vi "Minimal X410 (FPGA).vi"() -> ()   [LabVIEW 2023]
uses:
  <vilib>/Platform/TimedLoop/XDataNode/XDataNode.xnode
  <vilib>/Platform/TimedLoop/XDataNode/nitl_modes.ctl
  <vilib>/Platform/TimedLoop/XDataNode/XDNodeRunTimeDep.lvlib
  <vilib>/Platform/TimedLoop/XDataNode/wakeup.ctl
  <vilib>/Platform/TimedLoop/XDataNode/timing_clust.ctl
  <vilib>/eio/EIONode/EIONode.xnode
  <vilib>/rvi/eio/common/nirviEmuTemplateMethod_errors.vi
  <instrlib>/_niInstr/DSP/v1/Shared/Public/IQ Data.ctl
  <instrlib>/_niInstr/DSP/v1/FPGA/Public/Sub VIs/Data Conversion/I16 to IQ - 1 spc - S18.1.vi
  <instrlib>/niUSRP/Reference FPGA/Tx Core/niUSRP Tx Core v1 FPGA.lvclass
  <vilib>/rvi/DataTransferAndStorage/Container/XNode/niFpgaContainer.xnode
  <vilib>/rvi/FIFO/Fifo_Resource/niFpgaFifoEmulationRefIn.vi
panel:
  out "scratch reg value":u32
  in  "update scratch reg":bool
  in  "scratch reg new value":u32
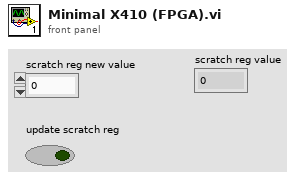
[diagram p1: front panel]
types:
  T1 = typedef "XDNodeRunTimeDep.lvlib/timing_clust.ctl" = cluster{"Expected End [f-1]":u64, "Actual End [f-1]":u64, "Finished Late? [f-1]":bool, "Expected End [i-1]":u64, "Actual End [i-1]":u64, "Finished Late? [i-1]":bool, "Expected Start [i]":u64, "Actual Start [i]":u64, "Expected Start [f]":u64, "Actual Start [f]":u64, "Source Name":string, "Structure Name":string, "Period":i64, "Deadline":i64, "Offset":i64, "Start":i64, "Priority":i32, "Timeout":i32, "Mode":T2, "Wakeup Reason":T3, "Error":errorcluster, "Source Type":string, "Secondary Source Type":string, "Global End Time":u64, "Global Start Time":u64, "Frame Duration":u64, "Iteration Duration":u64, "Assigned CPU":i32, "I/O Scan Engine Mode":u32}
  T2 = typedef "XDNodeRunTimeDep.lvlib/nitl_modes.ctl" = enum32{"No Change", "Process missed periods, maintain original phase", "Discard missed periods, maintain original phase", "Process missed periods, ignore original phase", "Discard missed periods, ignore original phase"}
  T3 = typedef "XDNodeRunTimeDep.lvlib/wakeup.ctl" = enum32{"Normal", "Aborted", "Asynchronous wakeup", "Timing source error", "Timed loop error", "Timeout"}
  T4 = typedef "niInstr DSP v1 Shared.lvlib/IQ Data.ctl" = cluster{"I":fxp<+/-,18,1>, "Q":fxp<+/-,18,1>, "overflow":bool}
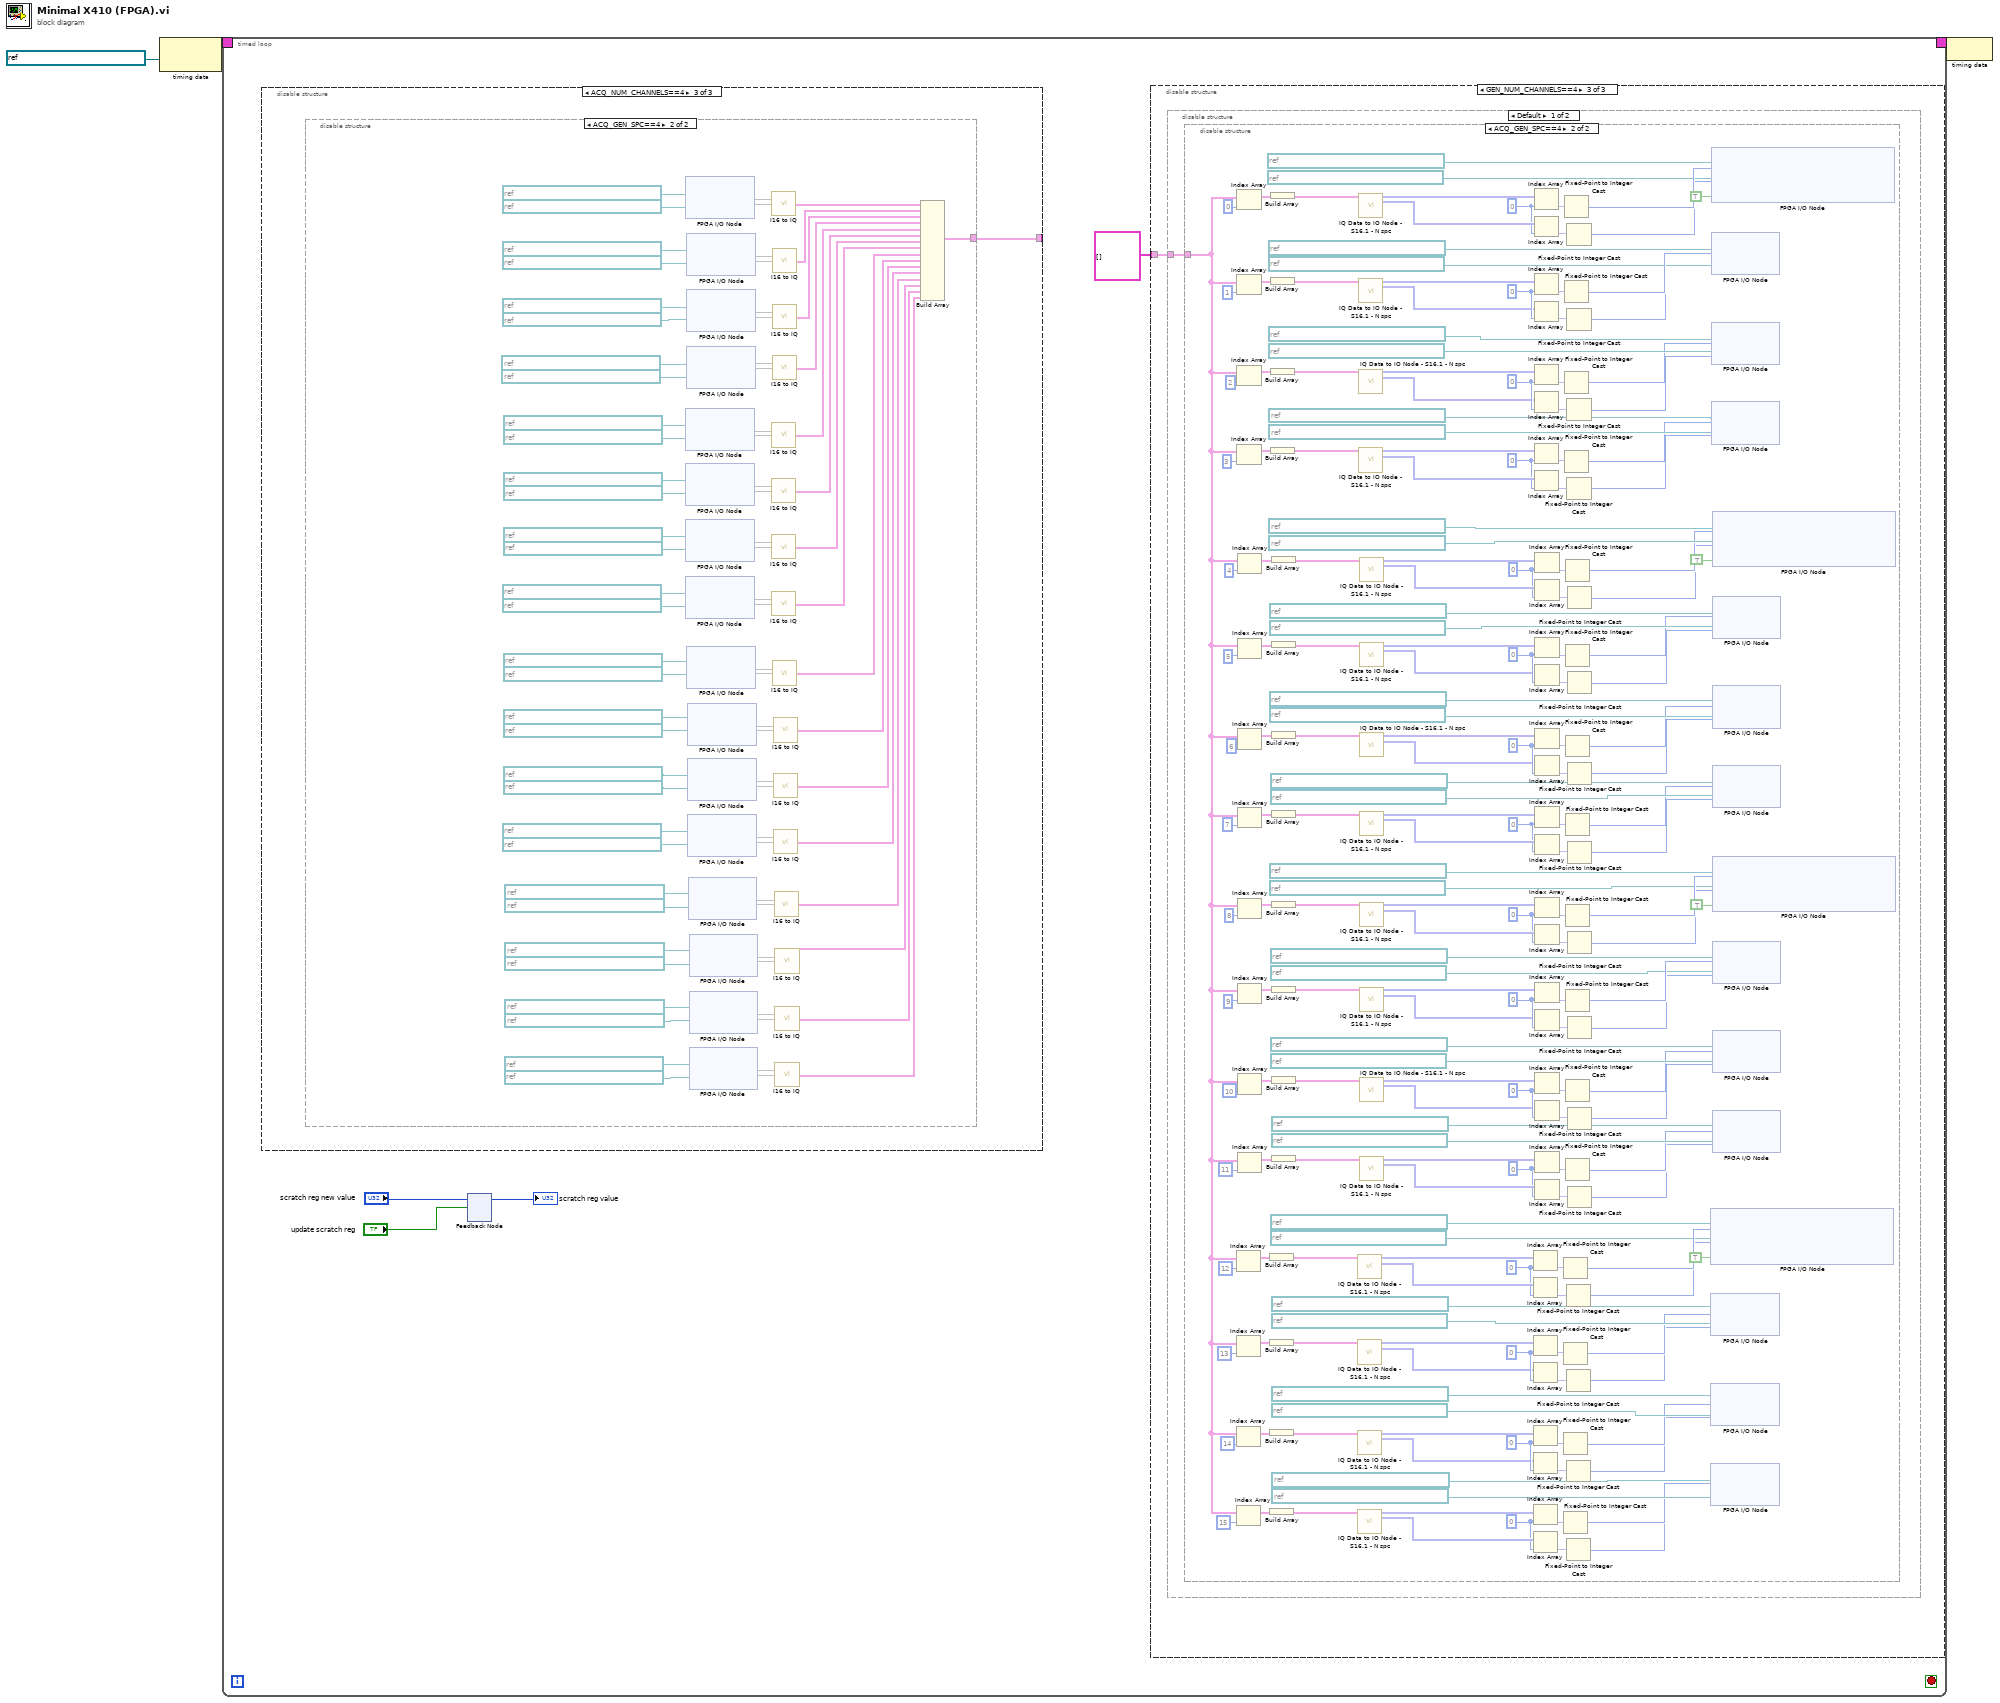
[diagram p0: block diagram]
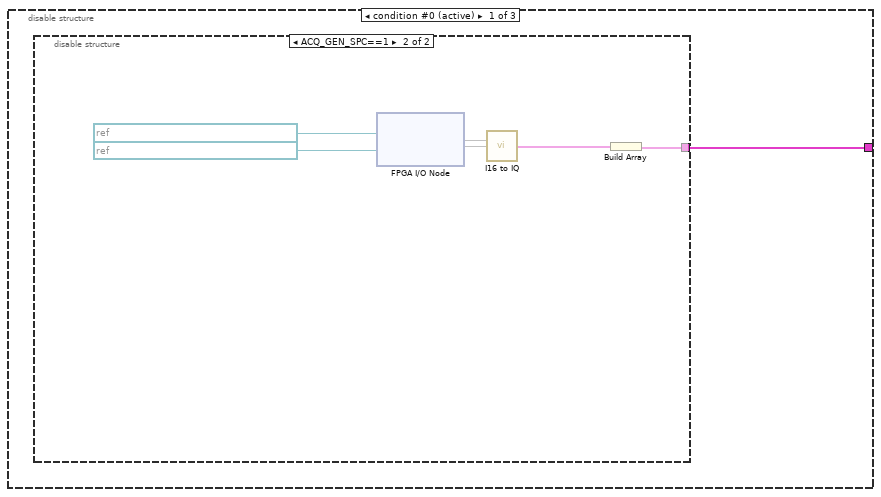
[diagram p2: hidden frame]
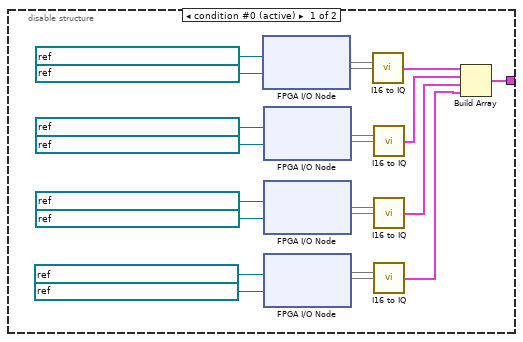
[diagram p3: hidden frame]
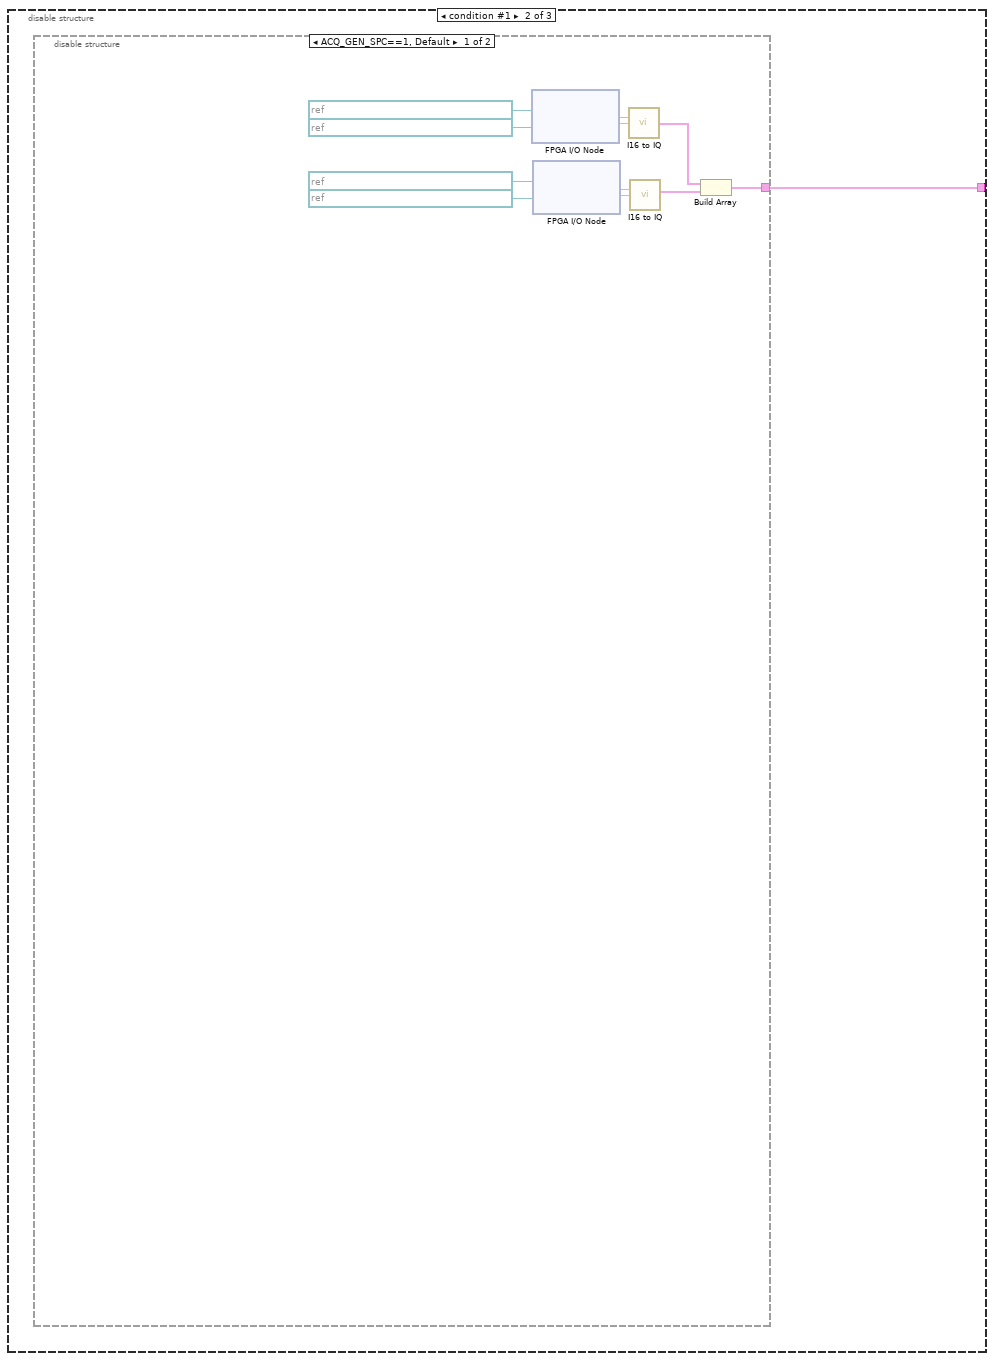
[diagram p4: hidden frame]
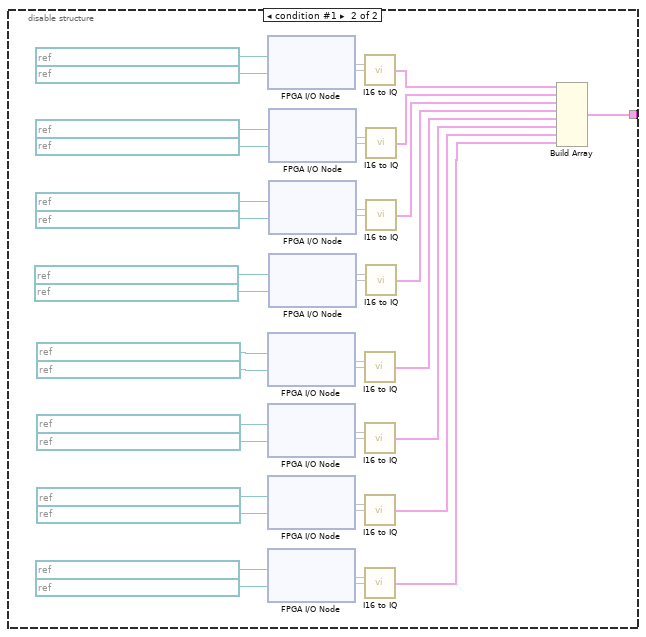
[diagram p5: hidden frame]
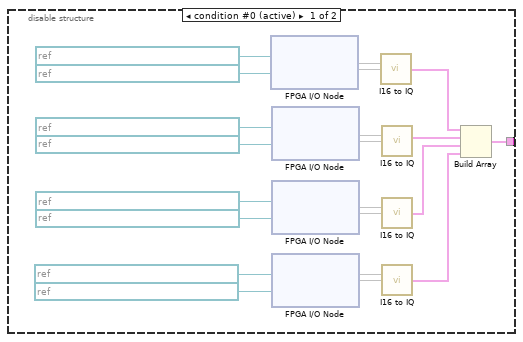
[diagram p6: hidden frame]
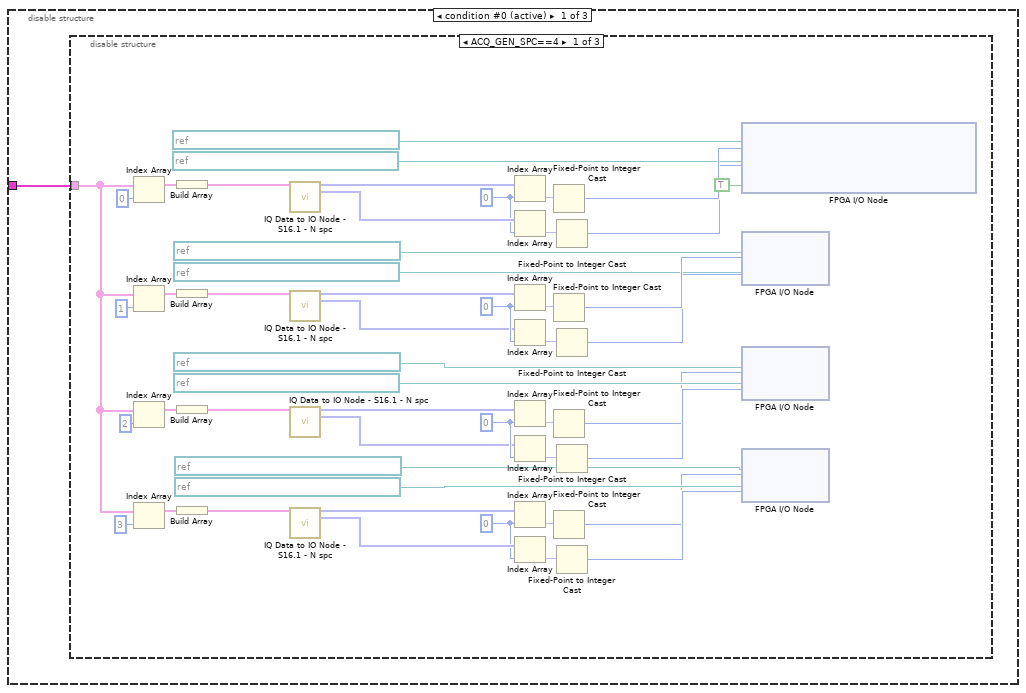
[diagram p7: hidden frame]
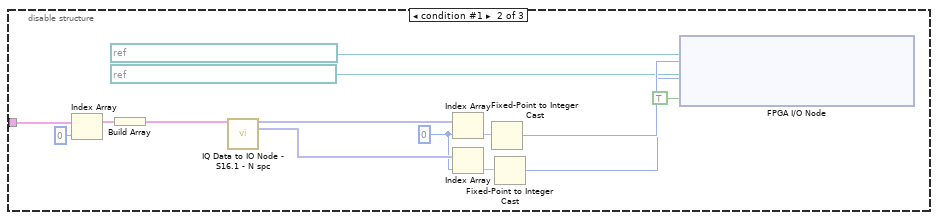
[diagram p8: hidden frame]
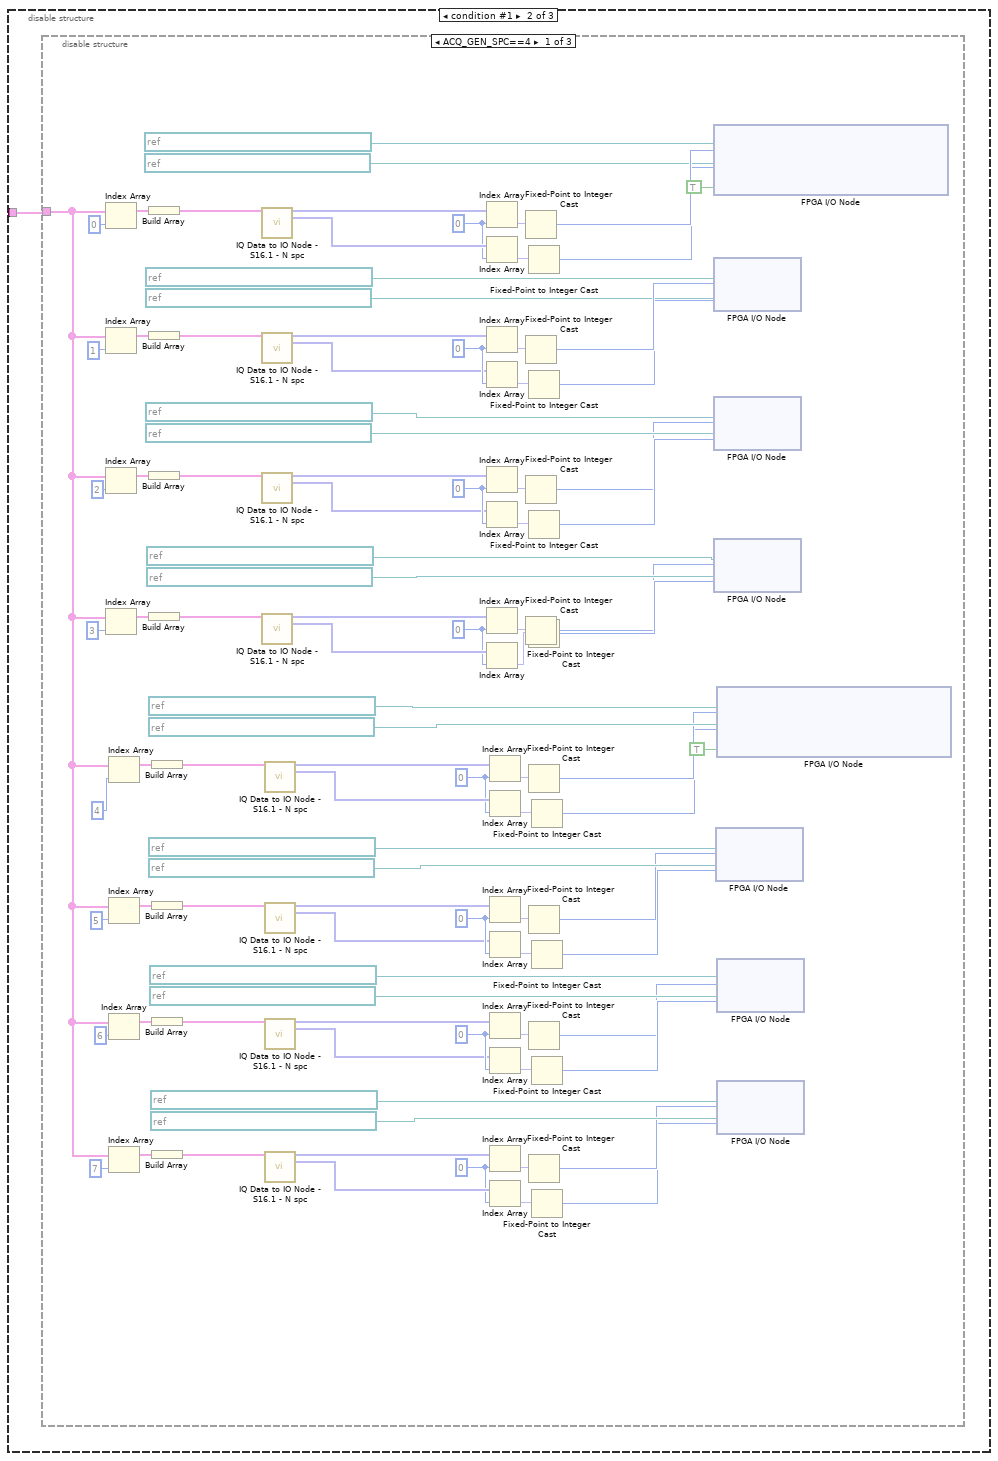
[diagram p10: hidden frame]
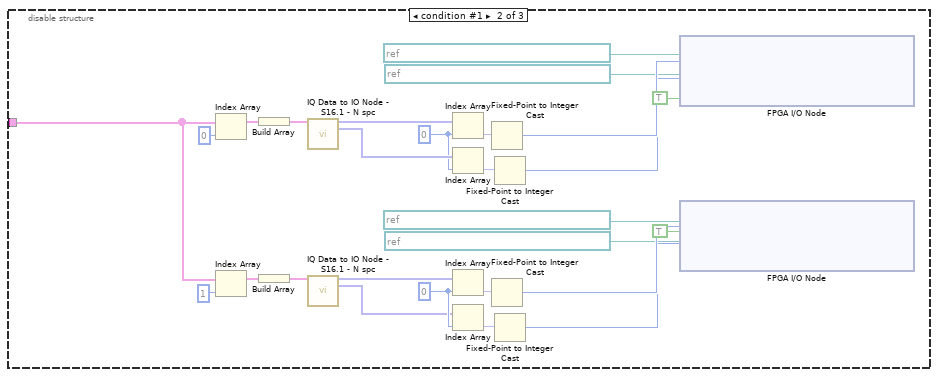
[diagram p11: hidden frame]
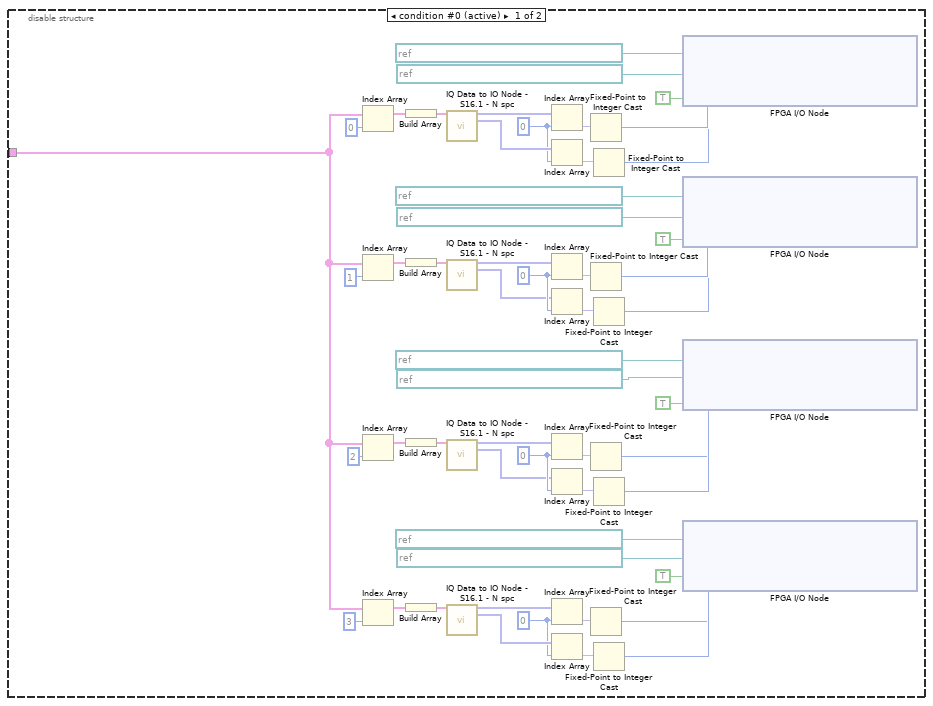
[diagram p13: hidden frame]
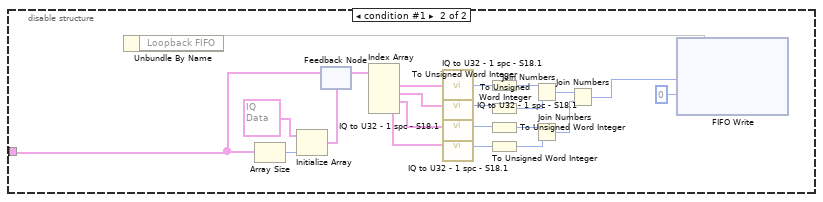
[diagram p14: hidden frame]
diagram:
  n1 = node-c288(refnum<k21> "Daughterboard 0\\Data Clock" ("Source Name")) -> (w3:T1)
  n2 = timed-loop {
    timing: w3 -> [_]
    timing-out: [_] -> w2
    stop <- _ stop-if-true
    n3 = disable-structure shown="ACQ_NUM_CHANNELS==4" {
      disable-tunnel: [w8 w36 w89] -> _
      frame condition #0 (active) {
        n4 = disable-structure shown="ACQ_GEN_SPC==1" {
          disable-tunnel: [w9 w35] -> w8
          frame condition #0 (active) {
            n5 = xnode "FPGA I/O Node"("FPGA I/O In"=refnum<k21> "Daughterboard 0\\RF 0\\Rx\\I0", "FPGA I/O In"=refnum<k21> "Daughterboard 0\\RF 0\\Rx\\Q0") -> ("I/O Item"=w29, "I/O Item"=w28)  [unwired: 2 out]
            n6 = xnode "FPGA I/O Node"("FPGA I/O In"=refnum<k21> "Daughterboard 0\\RF 0\\Rx\\I1", "FPGA I/O In"=refnum<k21> "Daughterboard 0\\RF 0\\Rx\\Q1") -> ("I/O Item"=w27, "I/O Item"=w26)  [unwired: 2 out]
            n7 = xnode "FPGA I/O Node"("FPGA I/O In"=refnum<k21> "Daughterboard 0\\RF 0\\Rx\\I2", "FPGA I/O In"=refnum<k21> "Daughterboard 0\\RF 0\\Rx\\Q2") -> ("I/O Item"=w25, "I/O Item"=w24)  [unwired: 2 out]
            n8 = xnode "FPGA I/O Node"("FPGA I/O In"=refnum<k21> "Daughterboard 0\\RF 0\\Rx\\I3", "FPGA I/O In"=refnum<k21> "Daughterboard 0\\RF 0\\Rx\\Q3") -> ("I/O Item"=w23, "I/O Item"=w22)  [unwired: 2 out]
            n9 = call-poly <instrlib>:"I16 to IQ.vi"("I"=w29, "Q"=w28) -> ("IQ"=w13:T4)  [unwired: 13 in]
            n10 = call-poly <instrlib>:"I16 to IQ.vi"("I"=w27, "Q"=w26) -> ("IQ"=w12:T4)  [unwired: 13 in]
            n11 = call-poly <instrlib>:"I16 to IQ.vi"("I"=w25, "Q"=w24) -> ("IQ"=w11:T4)  [unwired: 13 in]
            n12 = call-poly <instrlib>:"I16 to IQ.vi"("I"=w23, "Q"=w22) -> ("IQ"=w10:T4)  [unwired: 13 in]
            n13 = Build Array(w13, w12, w11, w10) -> (w9:T4[])
          }
          frame condition #1 {
            n14 = xnode "FPGA I/O Node"("FPGA I/O In"=refnum<k21> "Daughterboard 0\\RF 0\\Rx\\I", "FPGA I/O In"=refnum<k21> "Daughterboard 0\\RF 0\\Rx\\Q") -> ("I/O Item"=w34, "I/O Item"=w33)  [unwired: 2 out]
            n15 = call-poly <instrlib>:"I16 to IQ.vi"("I"=w34, "Q"=w33) -> ("IQ"=w30:T4)  [unwired: 13 in]
            n16 = Build Array(w30) -> (w35:T4[])
          }
        }
      }
      frame condition #1 {
        n17 = disable-structure shown="ACQ_GEN_SPC==1, Default" {
          disable-tunnel: [w37 w88] -> w36
          frame condition #0 (active) {
            n18 = xnode "FPGA I/O Node"("FPGA I/O In"=refnum<k21> "Daughterboard 0\\RF 0\\Rx\\I", "FPGA I/O In"=refnum<k21> "Daughterboard 0\\RF 0\\Rx\\Q") -> ("I/O Item"=w47, "I/O Item"=w46)  [unwired: 2 out]
            n19 = xnode "FPGA I/O Node"("FPGA I/O In"=refnum<k21> "Daughterboard 0\\RF 1\\Rx\\I", "FPGA I/O In"=refnum<k21> "Daughterboard 0\\RF 1\\Rx\\Q") -> ("I/O Item"=w45, "I/O Item"=w44)  [unwired: 2 out]
            n20 = call-poly <instrlib>:"I16 to IQ.vi"("I"=w47, "Q"=w46) -> ("IQ"=w39:T4)  [unwired: 13 in]
            n21 = call-poly <instrlib>:"I16 to IQ.vi"("I"=w45, "Q"=w44) -> ("IQ"=w38:T4)  [unwired: 13 in]
            n22 = Build Array(w39, w38) -> (w37:T4[])
          }
          frame condition #1 {
            n23 = xnode "FPGA I/O Node"("FPGA I/O In"=refnum<k21> "Daughterboard 0\\RF 0\\Rx\\I0", "FPGA I/O In"=refnum<k21> "Daughterboard 0\\RF 0\\Rx\\Q0") -> ("I/O Item"=w87, "I/O Item"=w86)  [unwired: 2 out]
            n24 = xnode "FPGA I/O Node"("FPGA I/O In"=refnum<k21> "Daughterboard 0\\RF 1\\Rx\\I0", "FPGA I/O In"=refnum<k21> "Daughterboard 0\\RF 1\\Rx\\Q0") -> ("I/O Item"=w78, "I/O Item"=w77)  [unwired: 2 out]
            n25 = xnode "FPGA I/O Node"("FPGA I/O In"=refnum<k21> "Daughterboard 0\\RF 1\\Rx\\I1", "FPGA I/O In"=refnum<k21> "Daughterboard 0\\RF 1\\Rx\\Q1") -> ("I/O Item"=w75, "I/O Item"=w74)  [unwired: 2 out]
            n26 = xnode "FPGA I/O Node"("FPGA I/O In"=refnum<k21> "Daughterboard 0\\RF 0\\Rx\\I2", "FPGA I/O In"=refnum<k21> "Daughterboard 0\\RF 1\\Rx\\Q2") -> ("I/O Item"=w73, "I/O Item"=w72)  [unwired: 2 out]
            n27 = xnode "FPGA I/O Node"("FPGA I/O In"=refnum<k21> "Daughterboard 0\\RF 1\\Rx\\I3", "FPGA I/O In"=refnum<k21> "Daughterboard 0\\RF 1\\Rx\\Q3") -> ("I/O Item"=w71, "I/O Item"=w70)  [unwired: 2 out]
            n28 = xnode "FPGA I/O Node"("FPGA I/O In"=refnum<k21> "Daughterboard 0\\RF 0\\Rx\\I1", "FPGA I/O In"=refnum<k21> "Daughterboard 0\\RF 0\\Rx\\Q1") -> ("I/O Item"=w84, "I/O Item"=w83)  [unwired: 2 out]
            n29 = xnode "FPGA I/O Node"("FPGA I/O In"=refnum<k21> "Daughterboard 0\\RF 0\\Rx\\I2", "FPGA I/O In"=refnum<k21> "Daughterboard 0\\RF 0\\Rx\\Q2") -> ("I/O Item"=w82, "I/O Item"=w81)  [unwired: 2 out]
            n30 = xnode "FPGA I/O Node"("FPGA I/O In"=refnum<k21> "Daughterboard 0\\RF 0\\Rx\\I3", "FPGA I/O In"=refnum<k21> "Daughterboard 0\\RF 0\\Rx\\Q3") -> ("I/O Item"=w80, "I/O Item"=w79)  [unwired: 2 out]
            n31 = call-poly <instrlib>:"I16 to IQ.vi"("I"=w87, "Q"=w86) -> ("IQ"=w85:T4)  [unwired: 13 in]
            n32 = call-poly <instrlib>:"I16 to IQ.vi"("I"=w78, "Q"=w77) -> ("IQ"=w76:T4)  [unwired: 13 in]
            n33 = call-poly <instrlib>:"I16 to IQ.vi"("I"=w75, "Q"=w74) -> ("IQ"=w66:T4)  [unwired: 13 in]
            n34 = call-poly <instrlib>:"I16 to IQ.vi"("I"=w73, "Q"=w72) -> ("IQ"=w65:T4)  [unwired: 13 in]
            n35 = call-poly <instrlib>:"I16 to IQ.vi"("I"=w71, "Q"=w70) -> ("IQ"=w64:T4)  [unwired: 13 in]
            n36 = call-poly <instrlib>:"I16 to IQ.vi"("I"=w84, "Q"=w83) -> ("IQ"=w69:T4)  [unwired: 13 in]
            n37 = call-poly <instrlib>:"I16 to IQ.vi"("I"=w82, "Q"=w81) -> ("IQ"=w68:T4)  [unwired: 13 in]
            n38 = call-poly <instrlib>:"I16 to IQ.vi"("I"=w80, "Q"=w79) -> ("IQ"=w67:T4)  [unwired: 13 in]
            n39 = Build Array(w85, w69, w68, w67, w76, w66, w65, w64) -> (w88:T4[])
          }
        }
      }
      frame condition #2 {
        n40 = disable-structure shown="ACQ_GEN_SPC==4" {
          disable-tunnel: [w90 w191] -> w89
          frame condition #0 (active) {
            n41 = xnode "FPGA I/O Node"("FPGA I/O In"=refnum<k21> "Daughterboard 0\\RF 0\\Rx\\I", "FPGA I/O In"=refnum<k21> "Daughterboard 0\\RF 0\\Rx\\Q") -> ("I/O Item"=w110, "I/O Item"=w109)  [unwired: 2 out]
            n42 = xnode "FPGA I/O Node"("FPGA I/O In"=refnum<k21> "Daughterboard 0\\RF 1\\Rx\\I", "FPGA I/O In"=refnum<k21> "Daughterboard 0\\RF 1\\Rx\\Q") -> ("I/O Item"=w108, "I/O Item"=w107)  [unwired: 2 out]
            n43 = xnode "FPGA I/O Node"("FPGA I/O In"=refnum<k21> "Daughterboard 1\\RF 0\\Rx\\I", "FPGA I/O In"=refnum<k21> "Daughterboard 1\\RF 0\\Rx\\Q") -> ("I/O Item"=w106, "I/O Item"=w105)  [unwired: 2 out]
            n44 = xnode "FPGA I/O Node"("FPGA I/O In"=refnum<k21> "Daughterboard 1\\RF 1\\Rx\\I", "FPGA I/O In"=refnum<k21> "Daughterboard 1\\RF 1\\Rx\\Q") -> ("I/O Item"=w104, "I/O Item"=w103)  [unwired: 2 out]
            n45 = call-poly <instrlib>:"I16 to IQ.vi"("I"=w110, "Q"=w109) -> ("IQ"=w94:T4)  [unwired: 13 in]
            n46 = call-poly <instrlib>:"I16 to IQ.vi"("I"=w108, "Q"=w107) -> ("IQ"=w93:T4)  [unwired: 13 in]
            n47 = call-poly <instrlib>:"I16 to IQ.vi"("I"=w106, "Q"=w105) -> ("IQ"=w92:T4)  [unwired: 13 in]
            n48 = call-poly <instrlib>:"I16 to IQ.vi"("I"=w104, "Q"=w103) -> ("IQ"=w91:T4)  [unwired: 13 in]
            n49 = Build Array(w94, w93, w92, w91) -> (w90:T4[])
          }
          frame condition #1 {
            n50 = xnode "FPGA I/O Node"("FPGA I/O In"=refnum<k21> "Daughterboard 0\\RF 0\\Rx\\I0", "FPGA I/O In"=refnum<k21> "Daughterboard 0\\RF 0\\Rx\\Q0") -> ("I/O Item"=w190, "I/O Item"=w189)  [unwired: 2 out]
            n51 = xnode "FPGA I/O Node"("FPGA I/O In"=refnum<k21> "Daughterboard 0\\RF 1\\Rx\\I0", "FPGA I/O In"=refnum<k21> "Daughterboard 0\\RF 1\\Rx\\Q0") -> ("I/O Item"=w181, "I/O Item"=w180)  [unwired: 2 out]
            n52 = xnode "FPGA I/O Node"("FPGA I/O In"=refnum<k21> "Daughterboard 0\\RF 1\\Rx\\I1", "FPGA I/O In"=refnum<k21> "Daughterboard 0\\RF 1\\Rx\\Q1") -> ("I/O Item"=w178, "I/O Item"=w177)  [unwired: 2 out]
            n53 = xnode "FPGA I/O Node"("FPGA I/O In"=refnum<k21> "Daughterboard 0\\RF 1\\Rx\\I2", "FPGA I/O In"=refnum<k21> "Daughterboard 0\\RF 1\\Rx\\Q2") -> ("I/O Item"=w176, "I/O Item"=w175)  [unwired: 2 out]
            n54 = xnode "FPGA I/O Node"("FPGA I/O In"=refnum<k21> "Daughterboard 0\\RF 1\\Rx\\I3", "FPGA I/O In"=refnum<k21> "Daughterboard 0\\RF 1\\Rx\\Q3") -> ("I/O Item"=w174, "I/O Item"=w173)  [unwired: 2 out]
            n55 = xnode "FPGA I/O Node"("FPGA I/O In"=refnum<k21> "Daughterboard 0\\RF 0\\Rx\\I1", "FPGA I/O In"=refnum<k21> "Daughterboard 0\\RF 0\\Rx\\Q1") -> ("I/O Item"=w187, "I/O Item"=w186)  [unwired: 2 out]
            n56 = xnode "FPGA I/O Node"("FPGA I/O In"=refnum<k21> "Daughterboard 0\\RF 0\\Rx\\I2", "FPGA I/O In"=refnum<k21> "Daughterboard 0\\RF 0\\Rx\\Q2") -> ("I/O Item"=w185, "I/O Item"=w184)  [unwired: 2 out]
            n57 = xnode "FPGA I/O Node"("FPGA I/O In"=refnum<k21> "Daughterboard 0\\RF 0\\Rx\\I3", "FPGA I/O In"=refnum<k21> "Daughterboard 0\\RF 0\\Rx\\Q3") -> ("I/O Item"=w183, "I/O Item"=w182)  [unwired: 2 out]
            n58 = xnode "FPGA I/O Node"("FPGA I/O In"=refnum<k21> "Daughterboard 1\\RF 0\\Rx\\I0", "FPGA I/O In"=refnum<k21> "Daughterboard 1\\RF 0\\Rx\\Q0") -> ("I/O Item"=w172, "I/O Item"=w171)  [unwired: 2 out]
            n59 = xnode "FPGA I/O Node"("FPGA I/O In"=refnum<k21> "Daughterboard 1\\RF 0\\Rx\\I1", "FPGA I/O In"=refnum<k21> "Daughterboard 1\\RF 0\\Rx\\Q1") -> ("I/O Item"=w170, "I/O Item"=w169)  [unwired: 2 out]
            n60 = xnode "FPGA I/O Node"("FPGA I/O In"=refnum<k21> "Daughterboard 1\\RF 0\\Rx\\I2", "FPGA I/O In"=refnum<k21> "Daughterboard 1\\RF 0\\Rx\\Q2") -> ("I/O Item"=w168, "I/O Item"=w167)  [unwired: 2 out]
            n61 = xnode "FPGA I/O Node"("FPGA I/O In"=refnum<k21> "Daughterboard 1\\RF 0\\Rx\\I3", "FPGA I/O In"=refnum<k21> "Daughterboard 1\\RF 0\\Rx\\Q3") -> ("I/O Item"=w166, "I/O Item"=w165)  [unwired: 2 out]
            n62 = xnode "FPGA I/O Node"("FPGA I/O In"=refnum<k21> "Daughterboard 1\\RF 1\\Rx\\I0", "FPGA I/O In"=refnum<k21> "Daughterboard 1\\RF 1\\Rx\\Q0") -> ("I/O Item"=w164, "I/O Item"=w163)  [unwired: 2 out]
            n63 = xnode "FPGA I/O Node"("FPGA I/O In"=refnum<k21> "Daughterboard 1\\RF 1\\Rx\\I1", "FPGA I/O In"=refnum<k21> "Daughterboard 1\\RF 1\\Rx\\Q1") -> ("I/O Item"=w162, "I/O Item"=w161)  [unwired: 2 out]
            n64 = xnode "FPGA I/O Node"("FPGA I/O In"=refnum<k21> "Daughterboard 1\\RF 1\\Rx\\I2", "FPGA I/O In"=refnum<k21> "Daughterboard 1\\RF 1\\Rx\\Q2") -> ("I/O Item"=w160, "I/O Item"=w159)  [unwired: 2 out]
            n65 = xnode "FPGA I/O Node"("FPGA I/O In"=refnum<k21> "Daughterboard 1\\RF 1\\Rx\\I3", "FPGA I/O In"=refnum<k21> "Daughterboard 1\\RF 1\\Rx\\Q3") -> ("I/O Item"=w158, "I/O Item"=w140)  [unwired: 2 out]
            n66 = call-poly <instrlib>:"I16 to IQ.vi"("I"=w190, "Q"=w189) -> ("IQ"=w188:T4)  [unwired: 13 in]
            n67 = call-poly <instrlib>:"I16 to IQ.vi"("I"=w181, "Q"=w180) -> ("IQ"=w179:T4)  [unwired: 13 in]
            n68 = call-poly <instrlib>:"I16 to IQ.vi"("I"=w178, "Q"=w177) -> ("IQ"=w153:T4)  [unwired: 13 in]
            n69 = call-poly <instrlib>:"I16 to IQ.vi"("I"=w176, "Q"=w175) -> ("IQ"=w152:T4)  [unwired: 13 in]
            n70 = call-poly <instrlib>:"I16 to IQ.vi"("I"=w174, "Q"=w173) -> ("IQ"=w151:T4)  [unwired: 13 in]
            n71 = call-poly <instrlib>:"I16 to IQ.vi"("I"=w187, "Q"=w186) -> ("IQ"=w156:T4)  [unwired: 13 in]
            n72 = call-poly <instrlib>:"I16 to IQ.vi"("I"=w185, "Q"=w184) -> ("IQ"=w155:T4)  [unwired: 13 in]
            n73 = call-poly <instrlib>:"I16 to IQ.vi"("I"=w183, "Q"=w182) -> ("IQ"=w154:T4)  [unwired: 13 in]
            n74 = call-poly <instrlib>:"I16 to IQ.vi"("I"=w172, "Q"=w171) -> ("IQ"=w157:T4)  [unwired: 13 in]
            n75 = call-poly <instrlib>:"I16 to IQ.vi"("I"=w170, "Q"=w169) -> ("IQ"=w150:T4)  [unwired: 13 in]
            n76 = call-poly <instrlib>:"I16 to IQ.vi"("I"=w168, "Q"=w167) -> ("IQ"=w149:T4)  [unwired: 13 in]
            n77 = call-poly <instrlib>:"I16 to IQ.vi"("I"=w166, "Q"=w165) -> ("IQ"=w148:T4)  [unwired: 13 in]
            n78 = call-poly <instrlib>:"I16 to IQ.vi"("I"=w164, "Q"=w163) -> ("IQ"=w147:T4)  [unwired: 13 in]
            n79 = call-poly <instrlib>:"I16 to IQ.vi"("I"=w162, "Q"=w161) -> ("IQ"=w146:T4)  [unwired: 13 in]
            n80 = call-poly <instrlib>:"I16 to IQ.vi"("I"=w160, "Q"=w159) -> ("IQ"=w145:T4)  [unwired: 13 in]
            n81 = call-poly <instrlib>:"I16 to IQ.vi"("I"=w158, "Q"=w140) -> ("IQ"=w144:T4)  [unwired: 13 in]
            n82 = Build Array(w188, w156, w155, w154, w179, w153, w152, w151, w157, w150, w149, w148, w147, w146, w145, w144) -> (w191:T4[])
          }
        }
      }
    }
    n83 = feedback-in #1("scratch reg new value", "update scratch reg") -> ()
    n84 = feedback #1() -> (→"scratch reg value":u32)  [unwired: 1 in]
    n85 = disable-structure shown="GEN_NUM_CHANNELS==4" {
      disable-tunnel: T4[] [] ("data") -> [w192 w257 w384]
      frame condition #0 (active) {
        n86 = disable-structure shown="ACQ_GEN_SPC==4" {
          disable-tunnel: w192 -> [w193 w243 _]
          frame condition #0 {
            w218 = 0 ("index")
            w209 = 0 ("index")
            w228 = 0 ("index")
            w237 = 0 ("index")
            n87 = Index Array(array=w193, index=0) -> (element=w234:T4)
            n88 = Index Array(array=w193, index=1) -> (element=w229:T4)
            n89 = Index Array(array=w193, index=2) -> (element=w211:T4)
            n90 = Index Array(array=w193, index=3) -> (element=w216:T4)
            n91 = Build Array(w234) -> (w232:T4[])
            n92 = Build Array(w229) -> (w231:T4[])
            n93 = Build Array(w211) -> (w213:T4[])
            n94 = Build Array(w216) -> (w214:T4[])
            n95 = call <instrlib>:"IQ Data to IO Node - S16.1 - N spc.vi"("data in"=w232) -> ("I out"=w242:fxp<+/-,16,1>[], "Q out"=w241:fxp<+/-,16,1>[])  [unwired: 12 in, 1 out]
            n96 = call <instrlib>:"IQ Data to IO Node - S16.1 - N spc.vi"("data in"=w231) -> ("I out"=w223:fxp<+/-,16,1>[], "Q out"=w224:fxp<+/-,16,1>[])  [unwired: 12 in, 1 out]
            n97 = call <instrlib>:"IQ Data to IO Node - S16.1 - N spc.vi"("data in"=w213) -> ("I out"=w205:fxp<+/-,16,1>[], "Q out"=w206:fxp<+/-,16,1>[])  [unwired: 12 in, 1 out]
            n98 = call <instrlib>:"IQ Data to IO Node - S16.1 - N spc.vi"("data in"=w214) -> ("I out"=w222:fxp<+/-,16,1>[], "Q out"=w221:fxp<+/-,16,1>[])  [unwired: 12 in, 1 out]
            n99 = Index Array(array=w242, index=w237) -> (element=w240:fxp<+/-,16,1>)
            n100 = Index Array(array=w241, index=w237) -> (element=w238:fxp<+/-,16,1>)
            n101 = Index Array(array=w223, index=w228) -> (element=w225:fxp<+/-,16,1>)
            n102 = Index Array(array=w224, index=w228) -> (element=w227:fxp<+/-,16,1>)
            n103 = Index Array(array=w205, index=w209) -> (element=w207:fxp<+/-,16,1>)
            n104 = Index Array(array=w206, index=w209) -> (element=w208:fxp<+/-,16,1>)
            n105 = Index Array(array=w222, index=w218) -> (element=w220:fxp<+/-,16,1>)
            n106 = Index Array(array=w221, index=w218) -> (element=w219:fxp<+/-,16,1>)
            n107 = Fixed-Point to Integer Cast(1:w240) -> (0:w239:i16)
            n108 = Fixed-Point to Integer Cast(1:w225) -> (0:w226:i16)
            n109 = Fixed-Point to Integer Cast(1:w207) -> (0:w194:i16)
            n110 = Fixed-Point to Integer Cast(1:w220) -> (0:w196:i16)
            n111 = Fixed-Point to Integer Cast(1:w238) -> (0:w236:i16)
            n112 = Fixed-Point to Integer Cast(1:w227) -> (0:w195:i16)
            n113 = Fixed-Point to Integer Cast(1:w208) -> (0:w210:i16)
            n114 = Fixed-Point to Integer Cast(1:w219) -> (0:w217:i16)
            n115 = xnode "FPGA I/O Node"("I/O Item"=w239, "FPGA I/O In"=refnum<k21> "Daughterboard 0\\RF 0\\Tx\\I0" ("FPGA I/O"), "I/O Item"=w236, "FPGA I/O In"=refnum<k21> "Daughterboard 0\\RF 0\\Tx\\Q0" ("FPGA I/O"), "Daughterboard 0\\RF 0\\Tx\\Data Valid"=TRUE ("Daughterboard 1\\s1TxDbaCh0DataValid")) -> ()  [unwired: 1 in, 3 out]
            n116 = xnode "FPGA I/O Node"("I/O Item"=w226, "FPGA I/O In"=refnum<k21> "Daughterboard 0\\RF 0\\Tx\\I1" ("FPGA I/O"), "I/O Item"=w195, "FPGA I/O In"=refnum<k21> "Daughterboard 0\\RF 0\\Tx\\Q1" ("FPGA I/O")) -> ()  [unwired: 2 out]
            n117 = xnode "FPGA I/O Node"("I/O Item"=w194, "FPGA I/O In"=refnum<k21> "Daughterboard 0\\RF 0\\Tx\\I2" ("FPGA I/O"), "I/O Item"=w210, "FPGA I/O In"=refnum<k21> "Daughterboard 0\\RF 0\\Tx\\Q2" ("FPGA I/O")) -> ()  [unwired: 2 out]
            n118 = xnode "FPGA I/O Node"("I/O Item"=w196, "FPGA I/O In"=refnum<k21> "Daughterboard 0\\RF 0\\Tx\\I3" ("FPGA I/O"), "I/O Item"=w217, "FPGA I/O In"=refnum<k21> "Daughterboard 0\\RF 0\\Tx\\Q3" ("FPGA I/O")) -> ()  [unwired: 2 out]
          }
          frame condition #1 {
            w251 = 0 ("index")
            n119 = Index Array(array=w243, index=0) -> (element=w248:T4)
            n120 = Build Array(w248) -> (w246:T4[])
            n121 = call <instrlib>:"IQ Data to IO Node - S16.1 - N spc.vi"("data in"=w246) -> ("I out"=w256:fxp<+/-,16,1>[], "Q out"=w255:fxp<+/-,16,1>[])  [unwired: 12 in, 1 out]
            n122 = Index Array(array=w256, index=w251) -> (element=w254:fxp<+/-,16,1>)
            n123 = Index Array(array=w255, index=w251) -> (element=w252:fxp<+/-,16,1>)
            n124 = Fixed-Point to Integer Cast(1:w254) -> (0:w253:i16)
            n125 = Fixed-Point to Integer Cast(1:w252) -> (0:w250:i16)
            n126 = xnode "FPGA I/O Node"("I/O Item"=w253, "FPGA I/O In"=refnum<k21> "Daughterboard 0\\Ch0TxDataI" ("FPGA I/O"), "I/O Item"=w250, "FPGA I/O In"=refnum<k21> "Daughterboard 0\\Ch0TxDataQ" ("FPGA I/O"), "Daughterboard 0\\RF 0\\Tx\\Data Valid"=TRUE ("Daughterboard 1\\s1TxDbaCh0DataValid")) -> ()  [unwired: 1 in, 3 out]
          }
          frame condition #2 (active) {
          }
        }
      }
      frame condition #1 {
        n127 = disable-structure shown="ACQ_GEN_SPC==4" {
          disable-tunnel: w257 -> [w260 w357 _]
          frame condition #0 {
            w286 = 0 ("index")
            w278 = 0 ("index")
            w294 = 0 ("index")
            w303 = 0 ("index")
            w332 = 0 ("index")
            w323 = 0 ("index")
            w342 = 0 ("index")
            w351 = 0 ("index")
            n128 = Index Array(array=w260, index=0) -> (element=w348:T4)
            n129 = Index Array(array=w260, index=1) -> (element=w343:T4)
            n130 = Index Array(array=w260, index=2) -> (element=w325:T4)
            n131 = Index Array(array=w260, index=3) -> (element=w330:T4)
            n132 = Index Array(array=w260, index=4) -> (element=w301:T4)
            n133 = Index Array(array=w260, index=5) -> (element=w296:T4)
            n134 = Index Array(array=w260, index=6) -> (element=w280:T4)
            n135 = Index Array(array=w260, index=7) -> (element=w285:T4)
            n136 = Build Array(w348) -> (w346:T4[])
            n137 = Build Array(w343) -> (w345:T4[])
            n138 = Build Array(w325) -> (w327:T4[])
            n139 = Build Array(w330) -> (w328:T4[])
            n140 = Build Array(w301) -> (w299:T4[])
            n141 = Build Array(w296) -> (w298:T4[])
            n142 = Build Array(w280) -> (w282:T4[])
            n143 = Build Array(w285) -> (w283:T4[])
            n144 = call <instrlib>:"IQ Data to IO Node - S16.1 - N spc.vi"("data in"=w346) -> ("I out"=w356:fxp<+/-,16,1>[], "Q out"=w355:fxp<+/-,16,1>[])  [unwired: 12 in, 1 out]
            n145 = call <instrlib>:"IQ Data to IO Node - S16.1 - N spc.vi"("data in"=w345) -> ("I out"=w337:fxp<+/-,16,1>[], "Q out"=w338:fxp<+/-,16,1>[])  [unwired: 12 in, 1 out]
            n146 = call <instrlib>:"IQ Data to IO Node - S16.1 - N spc.vi"("data in"=w327) -> ("I out"=w319:fxp<+/-,16,1>[], "Q out"=w320:fxp<+/-,16,1>[])  [unwired: 12 in, 1 out]
            n147 = call <instrlib>:"IQ Data to IO Node - S16.1 - N spc.vi"("data in"=w328) -> ("I out"=w336:fxp<+/-,16,1>[], "Q out"=w335:fxp<+/-,16,1>[])  [unwired: 12 in, 1 out]
            n148 = call <instrlib>:"IQ Data to IO Node - S16.1 - N spc.vi"("data in"=w299) -> ("I out"=w307:fxp<+/-,16,1>[], "Q out"=w306:fxp<+/-,16,1>[])  [unwired: 12 in, 1 out]
            n149 = call <instrlib>:"IQ Data to IO Node - S16.1 - N spc.vi"("data in"=w298) -> ("I out"=w290:fxp<+/-,16,1>[], "Q out"=w291:fxp<+/-,16,1>[])  [unwired: 12 in, 1 out]
            n150 = call <instrlib>:"IQ Data to IO Node - S16.1 - N spc.vi"("data in"=w282) -> ("I out"=w274:fxp<+/-,16,1>[], "Q out"=w275:fxp<+/-,16,1>[])  [unwired: 12 in, 1 out]
            n151 = call <instrlib>:"IQ Data to IO Node - S16.1 - N spc.vi"("data in"=w283) -> ("I out"=w289:fxp<+/-,16,1>[], "Q out"=w288:fxp<+/-,16,1>[])  [unwired: 12 in, 1 out]
            n152 = Index Array(array=w356, index=w351) -> (element=w354:fxp<+/-,16,1>)
            n153 = Index Array(array=w355, index=w351) -> (element=w352:fxp<+/-,16,1>)
            n154 = Index Array(array=w337, index=w342) -> (element=w339:fxp<+/-,16,1>)
            n155 = Index Array(array=w338, index=w342) -> (element=w341:fxp<+/-,16,1>)
            n156 = Index Array(array=w319, index=w323) -> (element=w321:fxp<+/-,16,1>)
            n157 = Index Array(array=w320, index=w323) -> (element=w322:fxp<+/-,16,1>)
            n158 = Index Array(array=w336, index=w332) -> (element=w334:fxp<+/-,16,1>)
            n159 = Index Array(array=w335, index=w332) -> (element=w333:fxp<+/-,16,1>)
            n160 = Index Array(array=w307, index=w303) -> (element=w305:fxp<+/-,16,1>)
            n161 = Index Array(array=w306, index=w303) -> (element=w304:fxp<+/-,16,1>)
            n162 = Index Array(array=w290, index=w294) -> (element=w292:fxp<+/-,16,1>)
            n163 = Index Array(array=w291, index=w294) -> (element=w293:fxp<+/-,16,1>)
            n164 = Index Array(array=w274, index=w278) -> (element=w276:fxp<+/-,16,1>)
            n165 = Index Array(array=w275, index=w278) -> (element=w277:fxp<+/-,16,1>)
            n166 = Index Array(array=w289, index=w286) -> (element=w287:fxp<+/-,16,1>)
            n167 = Index Array(array=w288, index=w286) -> (element=w259:fxp<+/-,16,1>)
            n168 = Fixed-Point to Integer Cast(1:w354) -> (0:w353:i16)
            n169 = Fixed-Point to Integer Cast(1:w339) -> (0:w340:i16)
            n170 = Fixed-Point to Integer Cast(1:w321) -> (0:w308:i16)
            n171 = Fixed-Point to Integer Cast(1:w334) -> (0:w310:i16)
            n172 = Fixed-Point to Integer Cast(1:w352) -> (0:w350:i16)
            n173 = Fixed-Point to Integer Cast(1:w341) -> (0:w309:i16)
            n174 = Fixed-Point to Integer Cast(1:w322) -> (0:w324:i16)
            n175 = Fixed-Point to Integer Cast(1:w333) -> (0:w331:i16)
            n176 = Fixed-Point to Integer Cast(1:w305) -> (0:w264:i16)
            n177 = Fixed-Point to Integer Cast(1:w292) -> (0:w262:i16)
            n178 = Fixed-Point to Integer Cast(1:w276) -> (0:w261:i16)
            n179 = Fixed-Point to Integer Cast(1:w287) -> (0:w265:i16)
            n180 = Fixed-Point to Integer Cast(1:w304) -> (0:w263:i16)
            n181 = Fixed-Point to Integer Cast(1:w293) -> (0:w295:i16)
            n182 = Fixed-Point to Integer Cast(1:w277) -> (0:w279:i16)
            n183 = Fixed-Point to Integer Cast(1:w259) -> (0:w258:i16)
            n184 = xnode "FPGA I/O Node"("I/O Item"=w353, "FPGA I/O In"=refnum<k21> "Daughterboard 0\\RF 0\\Tx\\I0" ("FPGA I/O"), "I/O Item"=w350, "FPGA I/O In"=refnum<k21> "Daughterboard 0\\RF 0\\Tx\\Q0" ("FPGA I/O"), "Daughterboard 0\\RF 0\\Tx\\Data Valid"=TRUE ("Daughterboard 1\\s1TxDbaCh0DataValid")) -> ()  [unwired: 1 in, 3 out]
            n185 = xnode "FPGA I/O Node"("I/O Item"=w340, "FPGA I/O In"=refnum<k21> "Daughterboard 0\\RF 0\\Tx\\I1" ("FPGA I/O"), "I/O Item"=w309, "FPGA I/O In"=refnum<k21> "Daughterboard 0\\RF 0\\Tx\\Q1" ("FPGA I/O")) -> ()  [unwired: 2 out]
            n186 = xnode "FPGA I/O Node"("I/O Item"=w308, "FPGA I/O In"=refnum<k21> "Daughterboard 0\\RF 0\\Tx\\I2" ("FPGA I/O"), "I/O Item"=w324, "FPGA I/O In"=refnum<k21> "Daughterboard 0\\RF 0\\Tx\\Q2" ("FPGA I/O")) -> ()  [unwired: 2 out]
            n187 = xnode "FPGA I/O Node"("I/O Item"=w310, "FPGA I/O In"=refnum<k21> "Daughterboard 0\\RF 0\\Tx\\I3" ("FPGA I/O"), "I/O Item"=w331, "FPGA I/O In"=refnum<k21> "Daughterboard 0\\RF 0\\Tx\\Q3" ("FPGA I/O")) -> ()  [unwired: 2 out]
            n188 = xnode "FPGA I/O Node"("I/O Item"=w262, "FPGA I/O In"=refnum<k21> "Daughterboard 0\\RF 1\\Tx\\I1" ("FPGA I/O"), "I/O Item"=w295, "FPGA I/O In"=refnum<k21> "Daughterboard 0\\RF 1\\Tx\\Q1" ("FPGA I/O")) -> ()  [unwired: 2 out]
            n189 = xnode "FPGA I/O Node"("I/O Item"=w264, "FPGA I/O In"=refnum<k21> "Daughterboard 0\\RF 1\\Tx\\I0" ("FPGA I/O"), "I/O Item"=w263, "FPGA I/O In"=refnum<k21> "Daughterboard 0\\RF 1\\Tx\\Q0" ("FPGA I/O"), "Daughterboard 0\\RF 1\\Tx\\Data Valid"=TRUE ("Daughterboard 1\\s1TxDbaCh0DataValid")) -> ()  [unwired: 1 in, 3 out]
            n190 = xnode "FPGA I/O Node"("I/O Item"=w261, "FPGA I/O In"=refnum<k21> "Daughterboard 0\\RF 1\\Tx\\I2" ("FPGA I/O"), "I/O Item"=w279, "FPGA I/O In"=refnum<k21> "Daughterboard 0\\RF 1\\Tx\\Q2" ("FPGA I/O")) -> ()  [unwired: 2 out]
            n191 = xnode "FPGA I/O Node"("I/O Item"=w265, "FPGA I/O In"=refnum<k21> "Daughterboard 0\\RF 1\\Tx\\I3" ("FPGA I/O"), "I/O Item"=w258, "FPGA I/O In"=refnum<k21> "Daughterboard 0\\RF 1\\Tx\\Q3" ("FPGA I/O")) -> ()  [unwired: 2 out]
          }
          frame condition #1 {
            w368 = 0 ("index")
            w378 = 0 ("index")
            n192 = Index Array(array=w357, index=0) -> (element=w375:T4)
            n193 = Index Array(array=w357, index=1) -> (element=w370:T4)
            n194 = Build Array(w375) -> (w373:T4[])
            n195 = Build Array(w370) -> (w372:T4[])
            n196 = call <instrlib>:"IQ Data to IO Node - S16.1 - N spc.vi"("data in"=w373) -> ("I out"=w383:fxp<+/-,16,1>[], "Q out"=w382:fxp<+/-,16,1>[])  [unwired: 12 in, 1 out]
            n197 = call <instrlib>:"IQ Data to IO Node - S16.1 - N spc.vi"("data in"=w372) -> ("I out"=w363:fxp<+/-,16,1>[], "Q out"=w364:fxp<+/-,16,1>[])  [unwired: 12 in, 1 out]
            n198 = Index Array(array=w383, index=w378) -> (element=w381:fxp<+/-,16,1>)
            n199 = Index Array(array=w382, index=w378) -> (element=w379:fxp<+/-,16,1>)
            n200 = Index Array(array=w363, index=w368) -> (element=w365:fxp<+/-,16,1>)
            n201 = Index Array(array=w364, index=w368) -> (element=w367:fxp<+/-,16,1>)
            n202 = Fixed-Point to Integer Cast(1:w381) -> (0:w380:i16)
            n203 = Fixed-Point to Integer Cast(1:w365) -> (0:w366:i16)
            n204 = Fixed-Point to Integer Cast(1:w379) -> (0:w377:i16)
            n205 = Fixed-Point to Integer Cast(1:w367) -> (0:w358:i16)
            n206 = xnode "FPGA I/O Node"("I/O Item"=w380, "FPGA I/O In"=refnum<k21> "Daughterboard 0\\RF 0\\Tx\\I" ("FPGA I/O"), "I/O Item"=w377, "FPGA I/O In"=refnum<k21> "Daughterboard 0\\RF 0\\Tx\\Q" ("FPGA I/O"), "Daughterboard 0\\RF 0\\Tx\\Data Valid"=TRUE ("Daughterboard 1\\s1TxDbaCh0DataValid")) -> ()  [unwired: 1 in, 3 out]
            n207 = xnode "FPGA I/O Node"("I/O Item"=w366, "FPGA I/O In"=refnum<k21> "Daughterboard 0\\RF 1\\Tx\\I" ("FPGA I/O"), "I/O Item"=w358, "FPGA I/O In"=refnum<k21> "Daughterboard 0\\RF 1\\Tx\\Q" ("FPGA I/O"), "Daughterboard 0\\RF 1\\Tx\\Data Valid"=TRUE ("Daughterboard 1\\s1TxDbaCh0DataValid")) -> ()  [unwired: 1 in, 3 out]
          }
          frame condition #2 (active) {
          }
        }
      }
      frame condition #2 {
        n208 = disable-structure shown="Default" {
          disable-tunnel: w384 -> [w385 w648]
          frame condition #0 (active) {
            n209 = disable-structure shown="ACQ_GEN_SPC==4" {
              disable-tunnel: w385 -> [w386 w490]
              frame condition #0 (active) {
                w413 = 0 ("index")
                w402 = 0 ("index")
                w423 = 0 ("index")
                w433 = 0 ("index")
                n210 = Index Array(array=w386, index=0) -> (element=w430:T4)
                n211 = Index Array(array=w386, index=1) -> (element=w425:T4)
                n212 = Index Array(array=w386, index=2) -> (element=w405:T4)
                n213 = Index Array(array=w386, index=3) -> (element=w410:T4)
                n214 = Build Array(w430) -> (w428:T4[])
                n215 = Build Array(w425) -> (w427:T4[])
                n216 = Build Array(w405) -> (w407:T4[])
                n217 = Build Array(w410) -> (w408:T4[])
                n218 = call <instrlib>:"IQ Data to IO Node - S16.1 - N spc.vi"("data in"=w428) -> ("I out"=w438:fxp<+/-,16,1>[], "Q out"=w437:fxp<+/-,16,1>[])  [unwired: 12 in, 1 out]
                n219 = call <instrlib>:"IQ Data to IO Node - S16.1 - N spc.vi"("data in"=w427) -> ("I out"=w418:fxp<+/-,16,1>[], "Q out"=w419:fxp<+/-,16,1>[])  [unwired: 12 in, 1 out]
                n220 = call <instrlib>:"IQ Data to IO Node - S16.1 - N spc.vi"("data in"=w407) -> ("I out"=w398:fxp<+/-,16,1>[], "Q out"=w399:fxp<+/-,16,1>[])  [unwired: 12 in, 1 out]
                n221 = call <instrlib>:"IQ Data to IO Node - S16.1 - N spc.vi"("data in"=w408) -> ("I out"=w417:fxp<+/-,16,1>[], "Q out"=w416:fxp<+/-,16,1>[])  [unwired: 12 in, 1 out]
                n222 = Index Array(array=w438, index=w433) -> (element=w436:fxp<+/-,16,1>)
                n223 = Index Array(array=w437, index=w433) -> (element=w434:fxp<+/-,16,1>)
                n224 = Index Array(array=w418, index=w423) -> (element=w420:fxp<+/-,16,1>)
                n225 = Index Array(array=w419, index=w423) -> (element=w422:fxp<+/-,16,1>)
                n226 = Index Array(array=w398, index=w402) -> (element=w400:fxp<+/-,16,1>)
                n227 = Index Array(array=w399, index=w402) -> (element=w401:fxp<+/-,16,1>)
                n228 = Index Array(array=w417, index=w413) -> (element=w415:fxp<+/-,16,1>)
                n229 = Index Array(array=w416, index=w413) -> (element=w414:fxp<+/-,16,1>)
                n230 = Fixed-Point to Integer Cast(1:w436) -> (0:w435:i16)
                n231 = Fixed-Point to Integer Cast(1:w420) -> (0:w421:i16)
                n232 = Fixed-Point to Integer Cast(1:w400) -> (0:w387:i16)
                n233 = Fixed-Point to Integer Cast(1:w415) -> (0:w389:i16)
                n234 = Fixed-Point to Integer Cast(1:w434) -> (0:w432:i16)
                n235 = Fixed-Point to Integer Cast(1:w422) -> (0:w388:i16)
                n236 = Fixed-Point to Integer Cast(1:w401) -> (0:w403:i16)
                n237 = Fixed-Point to Integer Cast(1:w414) -> (0:w412:i16)
                n238 = xnode "FPGA I/O Node"("I/O Item"=w435, "FPGA I/O In"=refnum<k21> "Daughterboard 0\\RF 0\\Tx\\I" ("FPGA I/O"), "I/O Item"=w432, "FPGA I/O In"=refnum<k21> "Daughterboard 0\\RF 0\\Tx\\Q" ("FPGA I/O"), "Daughterboard 0\\RF 0\\Tx\\Data Valid"=TRUE ("Daughterboard 1\\s1TxDbaCh0DataValid")) -> ()  [unwired: 1 in, 3 out]
                n239 = xnode "FPGA I/O Node"("I/O Item"=w421, "FPGA I/O In"=refnum<k21> "Daughterboard 0\\RF 1\\Tx\\I" ("FPGA I/O"), "I/O Item"=w388, "FPGA I/O In"=refnum<k21> "Daughterboard 0\\RF 1\\Tx\\Q" ("FPGA I/O"), "Daughterboard 0\\RF 1\\Tx\\Data Valid"=TRUE ("Daughterboard 1\\s1TxDbaCh0DataValid")) -> ()  [unwired: 1 in, 3 out]
                n240 = xnode "FPGA I/O Node"("I/O Item"=w387, "FPGA I/O In"=refnum<k21> "Daughterboard 1\\RF 0\\Tx\\I" ("FPGA I/O"), "I/O Item"=w403, "FPGA I/O In"=refnum<k21> "Daughterboard 1\\RF 0\\Tx\\Q" ("FPGA I/O"), "Daughterboard 1\\RF 0\\Tx\\Data Valid"=TRUE ("Daughterboard 1\\s1TxDbaCh0DataValid")) -> ()  [unwired: 1 in, 3 out]
                n241 = xnode "FPGA I/O Node"("I/O Item"=w389, "FPGA I/O In"=refnum<k21> "Daughterboard 1\\RF 1\\Tx\\I" ("FPGA I/O"), "I/O Item"=w412, "FPGA I/O In"=refnum<k21> "Daughterboard 1\\RF 1\\Tx\\Q" ("FPGA I/O"), "Daughterboard 1\\RF 1\\Tx\\Data Valid"=TRUE ("Daughterboard 1\\s1TxDbaCh0DataValid")) -> ()  [unwired: 1 in, 3 out]
              }
              frame condition #1 {
                w502 = 0 ("index")
                w495 = 0 ("index")
                w511 = 0 ("index")
                w520 = 0 ("index")
                w537 = 0 ("index")
                w530 = 0 ("index")
                w547 = 0 ("index")
                w556 = 0 ("index")
                w575 = 0 ("index")
                w566 = 0 ("index")
                w584 = 0 ("index")
                w593 = 0 ("index")
                w611 = 0 ("index")
                w602 = 0 ("index")
                w621 = 0 ("index")
                w630 = 0 ("index")
                n242 = Index Array(array=w490, index=12) -> (element=w517:T4)
                n243 = Index Array(array=w490, index=13) -> (element=w512:T4)
                n244 = Index Array(array=w490, index=14) -> (element=w496:T4)
                n245 = Index Array(array=w490, index=15) -> (element=w501:T4)
                n246 = Index Array(array=w490, index=0) -> (element=w627:T4)
                n247 = Index Array(array=w490, index=1) -> (element=w622:T4)
                n248 = Index Array(array=w490, index=2) -> (element=w604:T4)
                n249 = Index Array(array=w490, index=3) -> (element=w609:T4)
                n250 = Index Array(array=w490, index=4) -> (element=w591:T4)
                n251 = Index Array(array=w490, index=5) -> (element=w586:T4)
                n252 = Index Array(array=w490, index=6) -> (element=w568:T4)
                n253 = Index Array(array=w490, index=7) -> (element=w573:T4)
                n254 = Index Array(array=w490, index=8) -> (element=w553:T4)
                n255 = Index Array(array=w490, index=9) -> (element=w548:T4)
                n256 = Index Array(array=w490, index=10) -> (element=w531:T4)
                n257 = Index Array(array=w490, index=11) -> (element=w536:T4)
                n258 = Build Array(w517) -> (w515:T4[])
                n259 = Build Array(w512) -> (w514:T4[])
                n260 = Build Array(w496) -> (w498:T4[])
                n261 = Build Array(w501) -> (w499:T4[])
                n262 = Build Array(w627) -> (w625:T4[])
                n263 = Build Array(w622) -> (w624:T4[])
                n264 = Build Array(w604) -> (w606:T4[])
                n265 = Build Array(w609) -> (w607:T4[])
                n266 = Build Array(w591) -> (w589:T4[])
                n267 = Build Array(w586) -> (w588:T4[])
                n268 = Build Array(w568) -> (w570:T4[])
                n269 = Build Array(w573) -> (w571:T4[])
                n270 = Build Array(w553) -> (w551:T4[])
                n271 = Build Array(w548) -> (w550:T4[])
                n272 = Build Array(w531) -> (w533:T4[])
                n273 = Build Array(w536) -> (w534:T4[])
                n274 = call <instrlib>:"IQ Data to IO Node - S16.1 - N spc.vi"("data in"=w515) -> ("I out"=w525:fxp<+/-,16,1>[], "Q out"=w524:fxp<+/-,16,1>[])  [unwired: 12 in, 1 out]
                n275 = call <instrlib>:"IQ Data to IO Node - S16.1 - N spc.vi"("data in"=w514) -> ("I out"=w507:fxp<+/-,16,1>[], "Q out"=w508:fxp<+/-,16,1>[])  [unwired: 12 in, 1 out]
                n276 = call <instrlib>:"IQ Data to IO Node - S16.1 - N spc.vi"("data in"=w498) -> ("I out"=w491:fxp<+/-,16,1>[], "Q out"=w492:fxp<+/-,16,1>[])  [unwired: 12 in, 1 out]
                n277 = call <instrlib>:"IQ Data to IO Node - S16.1 - N spc.vi"("data in"=w499) -> ("I out"=w506:fxp<+/-,16,1>[], "Q out"=w505:fxp<+/-,16,1>[])  [unwired: 12 in, 1 out]
                n278 = call <instrlib>:"IQ Data to IO Node - S16.1 - N spc.vi"("data in"=w625) -> ("I out"=w635:fxp<+/-,16,1>[], "Q out"=w634:fxp<+/-,16,1>[])  [unwired: 12 in, 1 out]
                n279 = call <instrlib>:"IQ Data to IO Node - S16.1 - N spc.vi"("data in"=w624) -> ("I out"=w616:fxp<+/-,16,1>[], "Q out"=w617:fxp<+/-,16,1>[])  [unwired: 12 in, 1 out]
                n280 = call <instrlib>:"IQ Data to IO Node - S16.1 - N spc.vi"("data in"=w606) -> ("I out"=w598:fxp<+/-,16,1>[], "Q out"=w599:fxp<+/-,16,1>[])  [unwired: 12 in, 1 out]
                n281 = call <instrlib>:"IQ Data to IO Node - S16.1 - N spc.vi"("data in"=w607) -> ("I out"=w615:fxp<+/-,16,1>[], "Q out"=w614:fxp<+/-,16,1>[])  [unwired: 12 in, 1 out]
                n282 = call <instrlib>:"IQ Data to IO Node - S16.1 - N spc.vi"("data in"=w589) -> ("I out"=w597:fxp<+/-,16,1>[], "Q out"=w596:fxp<+/-,16,1>[])  [unwired: 12 in, 1 out]
                n283 = call <instrlib>:"IQ Data to IO Node - S16.1 - N spc.vi"("data in"=w588) -> ("I out"=w580:fxp<+/-,16,1>[], "Q out"=w581:fxp<+/-,16,1>[])  [unwired: 12 in, 1 out]
                n284 = call <instrlib>:"IQ Data to IO Node - S16.1 - N spc.vi"("data in"=w570) -> ("I out"=w562:fxp<+/-,16,1>[], "Q out"=w563:fxp<+/-,16,1>[])  [unwired: 12 in, 1 out]
                n285 = call <instrlib>:"IQ Data to IO Node - S16.1 - N spc.vi"("data in"=w571) -> ("I out"=w579:fxp<+/-,16,1>[], "Q out"=w578:fxp<+/-,16,1>[])  [unwired: 12 in, 1 out]
                n286 = call <instrlib>:"IQ Data to IO Node - S16.1 - N spc.vi"("data in"=w551) -> ("I out"=w561:fxp<+/-,16,1>[], "Q out"=w560:fxp<+/-,16,1>[])  [unwired: 12 in, 1 out]
                n287 = call <instrlib>:"IQ Data to IO Node - S16.1 - N spc.vi"("data in"=w550) -> ("I out"=w542:fxp<+/-,16,1>[], "Q out"=w543:fxp<+/-,16,1>[])  [unwired: 12 in, 1 out]
                n288 = call <instrlib>:"IQ Data to IO Node - S16.1 - N spc.vi"("data in"=w533) -> ("I out"=w526:fxp<+/-,16,1>[], "Q out"=w527:fxp<+/-,16,1>[])  [unwired: 12 in, 1 out]
                n289 = call <instrlib>:"IQ Data to IO Node - S16.1 - N spc.vi"("data in"=w534) -> ("I out"=w541:fxp<+/-,16,1>[], "Q out"=w540:fxp<+/-,16,1>[])  [unwired: 12 in, 1 out]
                n290 = Index Array(array=w525, index=w520) -> (element=w523:fxp<+/-,16,1>)
                n291 = Index Array(array=w524, index=w520) -> (element=w521:fxp<+/-,16,1>)
                n292 = Index Array(array=w507, index=w511) -> (element=w509:fxp<+/-,16,1>)
                n293 = Index Array(array=w508, index=w511) -> (element=w510:fxp<+/-,16,1>)
                n294 = Index Array(array=w491, index=w495) -> (element=w493:fxp<+/-,16,1>)
                n295 = Index Array(array=w492, index=w495) -> (element=w494:fxp<+/-,16,1>)
                n296 = Index Array(array=w506, index=w502) -> (element=w504:fxp<+/-,16,1>)
                n297 = Index Array(array=w505, index=w502) -> (element=w503:fxp<+/-,16,1>)
                n298 = Index Array(array=w635, index=w630) -> (element=w633:fxp<+/-,16,1>)
                n299 = Index Array(array=w634, index=w630) -> (element=w631:fxp<+/-,16,1>)
                n300 = Index Array(array=w616, index=w621) -> (element=w618:fxp<+/-,16,1>)
                n301 = Index Array(array=w617, index=w621) -> (element=w620:fxp<+/-,16,1>)
                n302 = Index Array(array=w598, index=w602) -> (element=w600:fxp<+/-,16,1>)
                n303 = Index Array(array=w599, index=w602) -> (element=w601:fxp<+/-,16,1>)
                n304 = Index Array(array=w615, index=w611) -> (element=w613:fxp<+/-,16,1>)
                n305 = Index Array(array=w614, index=w611) -> (element=w612:fxp<+/-,16,1>)
                n306 = Index Array(array=w597, index=w593) -> (element=w595:fxp<+/-,16,1>)
                n307 = Index Array(array=w596, index=w593) -> (element=w594:fxp<+/-,16,1>)
                n308 = Index Array(array=w580, index=w584) -> (element=w582:fxp<+/-,16,1>)
                n309 = Index Array(array=w581, index=w584) -> (element=w583:fxp<+/-,16,1>)
                n310 = Index Array(array=w562, index=w566) -> (element=w564:fxp<+/-,16,1>)
                n311 = Index Array(array=w563, index=w566) -> (element=w565:fxp<+/-,16,1>)
                n312 = Index Array(array=w579, index=w575) -> (element=w577:fxp<+/-,16,1>)
                n313 = Index Array(array=w578, index=w575) -> (element=w576:fxp<+/-,16,1>)
                n314 = Index Array(array=w561, index=w556) -> (element=w559:fxp<+/-,16,1>)
                n315 = Index Array(array=w560, index=w556) -> (element=w557:fxp<+/-,16,1>)
                n316 = Index Array(array=w542, index=w547) -> (element=w544:fxp<+/-,16,1>)
                n317 = Index Array(array=w543, index=w547) -> (element=w546:fxp<+/-,16,1>)
                n318 = Index Array(array=w526, index=w530) -> (element=w528:fxp<+/-,16,1>)
                n319 = Index Array(array=w527, index=w530) -> (element=w529:fxp<+/-,16,1>)
                n320 = Index Array(array=w541, index=w537) -> (element=w539:fxp<+/-,16,1>)
                n321 = Index Array(array=w540, index=w537) -> (element=w538:fxp<+/-,16,1>)
                n322 = Fixed-Point to Integer Cast(1:w523) -> (0:w522:i16)
                n323 = Fixed-Point to Integer Cast(1:w509) -> (0:w456:i16)
                n324 = Fixed-Point to Integer Cast(1:w493) -> (0:w462:i16)
                n325 = Fixed-Point to Integer Cast(1:w504) -> (0:w466:i16)
                n326 = Fixed-Point to Integer Cast(1:w633) -> (0:w632:i16)
                n327 = Fixed-Point to Integer Cast(1:w618) -> (0:w619:i16)
                n328 = Fixed-Point to Integer Cast(1:w600) -> (0:w441:i16)
                n329 = Fixed-Point to Integer Cast(1:w613) -> (0:w443:i16)
                n330 = Fixed-Point to Integer Cast(1:w595) -> (0:w445:i16)
                n331 = Fixed-Point to Integer Cast(1:w582) -> (0:w440:i16)
                n332 = Fixed-Point to Integer Cast(1:w564) -> (0:w439:i16)
                n333 = Fixed-Point to Integer Cast(1:w577) -> (0:w446:i16)
                n334 = Fixed-Point to Integer Cast(1:w559) -> (0:w558:i16)
                n335 = Fixed-Point to Integer Cast(1:w544) -> (0:w545:i16)
                n336 = Fixed-Point to Integer Cast(1:w528) -> (0:w447:i16)
                n337 = Fixed-Point to Integer Cast(1:w539) -> (0:w450:i16)
                n338 = Fixed-Point to Integer Cast(1:w521) -> (0:w519:i16)
                n339 = Fixed-Point to Integer Cast(1:w510) -> (0:w455:i16)
                n340 = Fixed-Point to Integer Cast(1:w494) -> (0:w461:i16)
                n341 = Fixed-Point to Integer Cast(1:w503) -> (0:w465:i16)
                n342 = Fixed-Point to Integer Cast(1:w631) -> (0:w629:i16)
                n343 = Fixed-Point to Integer Cast(1:w620) -> (0:w442:i16)
                n344 = Fixed-Point to Integer Cast(1:w601) -> (0:w603:i16)
                n345 = Fixed-Point to Integer Cast(1:w612) -> (0:w610:i16)
                n346 = Fixed-Point to Integer Cast(1:w594) -> (0:w444:i16)
                n347 = Fixed-Point to Integer Cast(1:w583) -> (0:w585:i16)
                n348 = Fixed-Point to Integer Cast(1:w565) -> (0:w567:i16)
                n349 = Fixed-Point to Integer Cast(1:w576) -> (0:w574:i16)
                n350 = Fixed-Point to Integer Cast(1:w557) -> (0:w555:i16)
                n351 = Fixed-Point to Integer Cast(1:w546) -> (0:w469:i16)
                n352 = Fixed-Point to Integer Cast(1:w529) -> (0:w448:i16)
                n353 = Fixed-Point to Integer Cast(1:w538) -> (0:w449:i16)
                n354 = xnode "FPGA I/O Node"("I/O Item"=w522, "FPGA I/O In"=refnum<k21> "Daughterboard 1\\RF 1\\Tx\\I0" ("FPGA I/O"), "I/O Item"=w519, "FPGA I/O In"=refnum<k21> "Daughterboard 1\\RF 1\\Tx\\Q0" ("FPGA I/O"), "Daughterboard 1\\RF 1\\Tx\\Data Valid"=TRUE ("Daughterboard 1\\s1TxDbaCh0DataValid")) -> ()  [unwired: 1 in, 3 out]
                n355 = xnode "FPGA I/O Node"("I/O Item"=w456, "FPGA I/O In"=refnum<k21> "Daughterboard 1\\RF 1\\Tx\\I1" ("FPGA I/O"), "I/O Item"=w455, "FPGA I/O In"=refnum<k21> "Daughterboard 1\\RF 1\\Tx\\Q1" ("FPGA I/O")) -> ()  [unwired: 2 out]
                n356 = xnode "FPGA I/O Node"("I/O Item"=w462, "FPGA I/O In"=refnum<k21> "Daughterboard 1\\RF 1\\Tx\\I2" ("FPGA I/O"), "I/O Item"=w461, "FPGA I/O In"=refnum<k21> "Daughterboard 1\\RF 1\\Tx\\Q2" ("FPGA I/O")) -> ()  [unwired: 2 out]
                n357 = xnode "FPGA I/O Node"("I/O Item"=w466, "FPGA I/O In"=refnum<k21> "Daughterboard 1\\RF 1\\Tx\\I3" ("FPGA I/O"), "I/O Item"=w465, "FPGA I/O In"=refnum<k21> "Daughterboard 1\\RF 1\\Tx\\Q3" ("FPGA I/O")) -> ()  [unwired: 2 out]
                n358 = xnode "FPGA I/O Node"("I/O Item"=w632, "FPGA I/O In"=refnum<k21> "Daughterboard 0\\RF 0\\Tx\\I0" ("FPGA I/O"), "I/O Item"=w629, "FPGA I/O In"=refnum<k21> "Daughterboard 0\\RF 0\\Tx\\Q0" ("FPGA I/O"), "Daughterboard 0\\RF 0\\Tx\\Data Valid"=TRUE ("Daughterboard 1\\s1TxDbaCh0DataValid")) -> ()  [unwired: 1 in, 3 out]
                n359 = xnode "FPGA I/O Node"("I/O Item"=w619, "FPGA I/O In"=refnum<k21> "Daughterboard 0\\RF 0\\Tx\\I1" ("FPGA I/O"), "I/O Item"=w442, "FPGA I/O In"=refnum<k21> "Daughterboard 0\\RF 0\\Tx\\Q1" ("FPGA I/O")) -> ()  [unwired: 2 out]
                n360 = xnode "FPGA I/O Node"("I/O Item"=w441, "FPGA I/O In"=refnum<k21> "Daughterboard 0\\RF 0\\Tx\\I2" ("FPGA I/O"), "I/O Item"=w603, "FPGA I/O In"=refnum<k21> "Daughterboard 0\\RF 0\\Tx\\Q2" ("FPGA I/O")) -> ()  [unwired: 2 out]
                n361 = xnode "FPGA I/O Node"("I/O Item"=w443, "FPGA I/O In"=refnum<k21> "Daughterboard 0\\RF 0\\Tx\\I3" ("FPGA I/O"), "I/O Item"=w610, "FPGA I/O In"=refnum<k21> "Daughterboard 0\\RF 0\\Tx\\Q3" ("FPGA I/O")) -> ()  [unwired: 2 out]
                n362 = xnode "FPGA I/O Node"("I/O Item"=w445, "FPGA I/O In"=refnum<k21> "Daughterboard 0\\RF 1\\Tx\\I0" ("FPGA I/O"), "I/O Item"=w444, "FPGA I/O In"=refnum<k21> "Daughterboard 0\\RF 1\\Tx\\Q0" ("FPGA I/O"), "Daughterboard 0\\RF 1\\Tx\\Data Valid"=TRUE ("Daughterboard 1\\s1TxDbaCh0DataValid")) -> ()  [unwired: 1 in, 3 out]
                n363 = xnode "FPGA I/O Node"("I/O Item"=w440, "FPGA I/O In"=refnum<k21> "Daughterboard 0\\RF 1\\Tx\\I1" ("FPGA I/O"), "I/O Item"=w585, "FPGA I/O In"=refnum<k21> "Daughterboard 0\\RF 1\\Tx\\Q1" ("FPGA I/O")) -> ()  [unwired: 2 out]
                n364 = xnode "FPGA I/O Node"("I/O Item"=w439, "FPGA I/O In"=refnum<k21> "Daughterboard 0\\RF 1\\Tx\\I2" ("FPGA I/O"), "I/O Item"=w567, "FPGA I/O In"=refnum<k21> "Daughterboard 0\\RF 1\\Tx\\Q2" ("FPGA I/O")) -> ()  [unwired: 2 out]
                n365 = xnode "FPGA I/O Node"("I/O Item"=w446, "FPGA I/O In"=refnum<k21> "Daughterboard 0\\RF 1\\Tx\\I3" ("FPGA I/O"), "I/O Item"=w574, "FPGA I/O In"=refnum<k21> "Daughterboard 0\\RF 1\\Tx\\Q3" ("FPGA I/O")) -> ()  [unwired: 2 out]
                n366 = xnode "FPGA I/O Node"("I/O Item"=w558, "FPGA I/O In"=refnum<k21> "Daughterboard 1\\RF 0\\Tx\\I0" ("FPGA I/O"), "I/O Item"=w555, "FPGA I/O In"=refnum<k21> "Daughterboard 1\\RF 0\\Tx\\Q0" ("FPGA I/O"), "Daughterboard 1\\RF 0\\Tx\\Data Valid"=TRUE ("Daughterboard 1\\s1TxDbaCh0DataValid")) -> ()  [unwired: 1 in, 3 out]
                n367 = xnode "FPGA I/O Node"("I/O Item"=w545, "FPGA I/O In"=refnum<k21> "Daughterboard 1\\RF 0\\Tx\\I1" ("FPGA I/O"), "I/O Item"=w469, "FPGA I/O In"=refnum<k21> "Daughterboard 1\\RF 0\\Tx\\Q1" ("FPGA I/O")) -> ()  [unwired: 2 out]
                n368 = xnode "FPGA I/O Node"("I/O Item"=w447, "FPGA I/O In"=refnum<k21> "Daughterboard 1\\RF 0\\Tx\\I2" ("FPGA I/O"), "I/O Item"=w448, "FPGA I/O In"=refnum<k21> "Daughterboard 1\\RF 0\\Tx\\Q2" ("FPGA I/O")) -> ()  [unwired: 2 out]
                n369 = xnode "FPGA I/O Node"("I/O Item"=w450, "FPGA I/O In"=refnum<k21> "Daughterboard 1\\RF 0\\Tx\\I3" ("FPGA I/O"), "I/O Item"=w449, "FPGA I/O In"=refnum<k21> "Daughterboard 1\\RF 0\\Tx\\Q3" ("FPGA I/O")) -> ()  [unwired: 2 out]
              }
            }
          }
          frame condition #1 {
            n370 = Unbundle By Name() -> (w649:refnum<class "niUSRP Tx Core v1 FPGA.lvclass">, "Loopback FIFO"=w658)
            n371 = Array Size(array=w648) -> (size(s)=w657:i32)
            n372 = Initialize Array(T4 {"I"=0.0, "Q"=0.0, "overflow"=FALSE} ("data"), w657) -> (w655:T4[])
            n373 = feedback #2(w655) -> (w653:T4[])
            n374 = feedback-in #2(w648) -> ()
            n375 = Index Array(array=w653) -> (element #1=w652:T4, element #2=w651:T4, element #3=w647:T4, element #4=w646:T4)  [unwired: 4 in]
            n376 = call <instrlib>:"IQ to U32 - 1 spc - S18.1.vi"("IQ data"=w652) -> ("U32 data"=w650:u32)  [unwired: 13 in, 1 out]
            n377 = call <instrlib>:"IQ to U32 - 1 spc - S18.1.vi"("IQ data"=w651) -> ("U32 data"=w642:u32)  [unwired: 13 in, 1 out]
            n378 = call <instrlib>:"IQ to U32 - 1 spc - S18.1.vi"("IQ data"=w647) -> ("U32 data"=w641:u32)  [unwired: 13 in, 1 out]
            n379 = call <instrlib>:"IQ to U32 - 1 spc - S18.1.vi"("IQ data"=w646) -> ("U32 data"=w640:u32)  [unwired: 13 in, 1 out]
            n380 = To Unsigned Word Integer(number=w650) -> (unsigned 16bit integer=w643:u16)
            n381 = To Unsigned Word Integer(number=w642) -> (unsigned 16bit integer=w639:u16)
            n382 = To Unsigned Word Integer(number=w641) -> (unsigned 16bit integer=w638:u16)
            n383 = To Unsigned Word Integer(number=w640) -> (unsigned 16bit integer=w637:u16)
            n384 = Join Numbers(hi=w643, lo=w639) -> ((hi.lo)=w645:u32)
            n385 = Join Numbers(hi=w638, lo=w637) -> ((hi.lo)=w636:u32)
            n386 = Join Numbers(hi=w645, lo=w636) -> ((hi.lo)=w644:u64)
            n387 = xnode ("FIFO Write")("Element"=w644, "Timeout"=0, "FIFO In"=w658) -> ()  [unwired: 2 out]
          }
        }
      }
    }
  }
  n388 = node-c288(w2) -> ()
